vi "Write prev_sequencia.vi"(8 "error in (no error)":errorcluster, 10 "prev_sequencia":u16, 11 "Opt_Selector in":refnum<class "Opt_Selector.lvclass">) -> (0 "error out":errorcluster, 3 "Opt_Selector out":refnum<class "Opt_Selector.lvclass">)   [LabVIEW 2018, in "Opt_Selector.lvclass"]
uses:
  Opt_Selector.lvclass
  Opt_Selector.lvclass/Opt_Selector.ctl
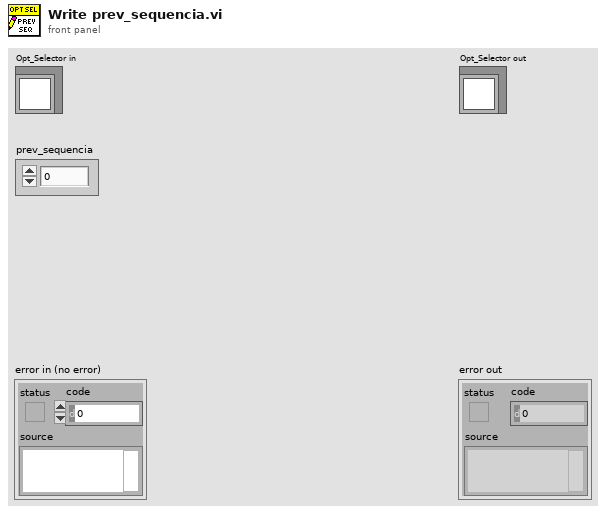
[diagram p1: front panel]
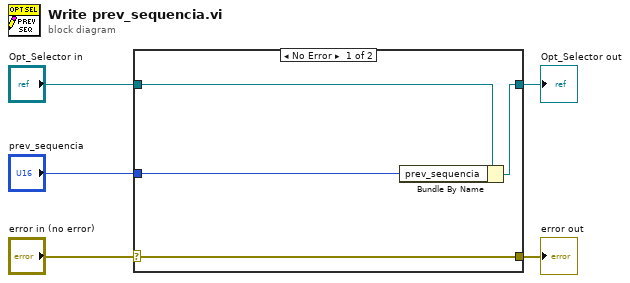
[diagram p0: block diagram]
diagram:
  n1 = case shown="No Error" "error in (no error)" {
    selector: "error in (no error)" -> [w9 w10]
    tunnel: [w9 w10] -> w4
    tunnel: [w7 w11] -> w2
    tunnel: "Opt_Selector in" -> [w8 w11]
    tunnel: "prev_sequencia" -> [w6 _]
    frame No Error {
      n2 = Bundle By Name(cluster=w8, "prev_sequencia"=w6) -> (w7:refnum<class "Opt_Selector.lvclass">)
    }
    frame Error {
    }
  }
  "error out" <- w4
  "Opt_Selector out" <- w2
